vi "Teardown.vi"(8 "Error in":errorcluster, 9 "Teardown Location":T1, 10 "Unheard Msgs":refnum<class "Message.lvclass">[](array[class]), 11 "TEMPLATE Actor in":refnum<class "{{Name}}Actor.lvclass">) -> (3 "TEMPLATE Actor out":refnum<class "{{Name}}Actor.lvclass">)   [LabVIEW 2020, in "_Template.lvlib" / "Templates.lvlib" / "{{Name}}Actor.lvlib" / "{{Name}}Actor.lvclass"]
uses:
  {{Name}}Actor.lvclass
  {{Name}}Actor.lvclass/{{Name}}Actor.ctl
  jettl/jettl/Message/Message.lvclass
  jettl/jettl/Actor/Actor.lvclass
  jettl/jettl/Teardown Location.ctl
  jettl/jettl/jettl.lvlib
panel:
  # "This front panel should not be manipulated."
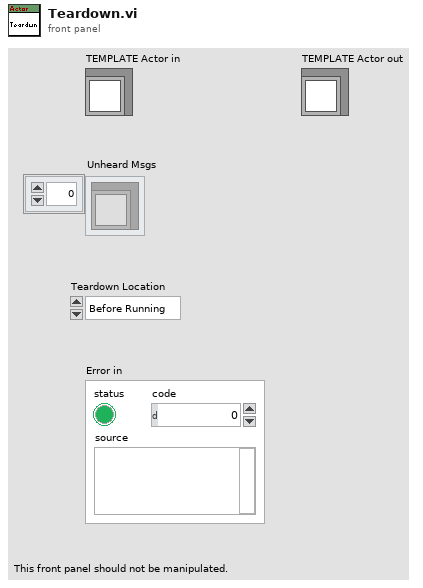
[diagram p1: front panel]
types:
  T1 = typedef "jettl.lvlib/Teardown Location.ctl" = enum16{"Before Running", "After Running"}
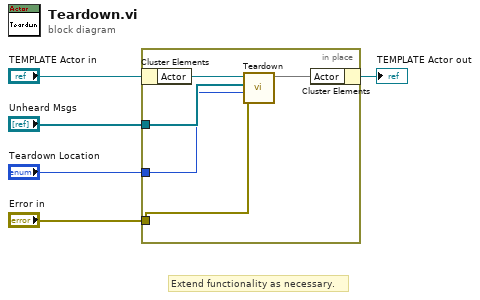
[diagram p0: block diagram]
diagram:
  # "Extend functionality as necessary."
  n1 = in-place {
    in-place-border: "Unheard Msgs" -> [w8]
    in-place-border: "Teardown Location" -> [w7]
    in-place-border: "Error in" -> [w6]
    n2 = in-place-cluster #1("TEMPLATE Actor in") -> ("Actor"=w10:refnum<class "Actor.lvclass">)
    n3 = call-dynamic "Teardown.vi"(8:w6, 9:w7, "Teardown Location"=w8, "Unheard Messages"=w10) -> (3:w9)  [unwired: 6 in, 1 out]
    n4 = in-place-cluster #1("Actor"=w9) -> (→"TEMPLATE Actor out":refnum<class "{{Name}}Actor.lvclass">)
  }
